vi "display.vi"(8 "error in (no error)":errorcluster, 11 "GeneralDisplay in":refnum<class "GeneralDisplay.lvclass">) -> (0 "error out":errorcluster, 3 "GeneralDisplay out":refnum<class "GeneralDisplay.lvclass">)   [LabVIEW 2018, in "GeneralDisplay.lvclass"]
uses:
  GeneralDisplay.lvclass
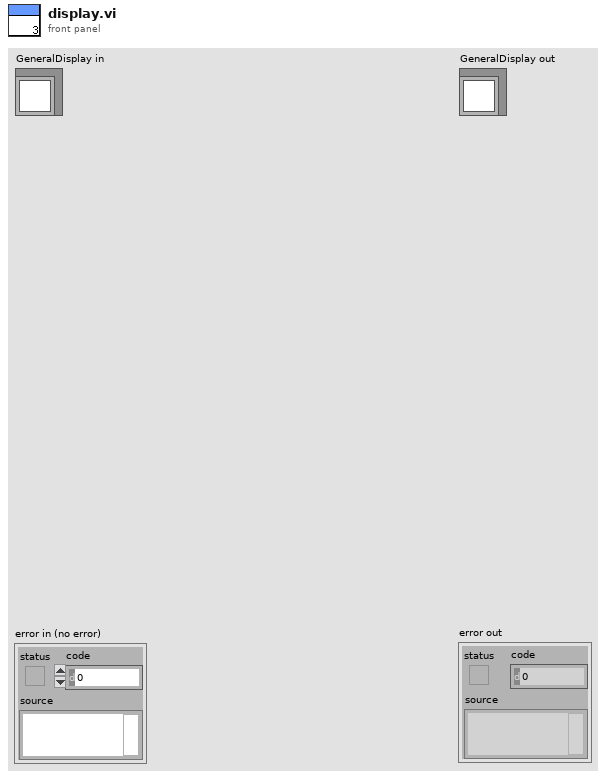
[diagram p1: front panel]
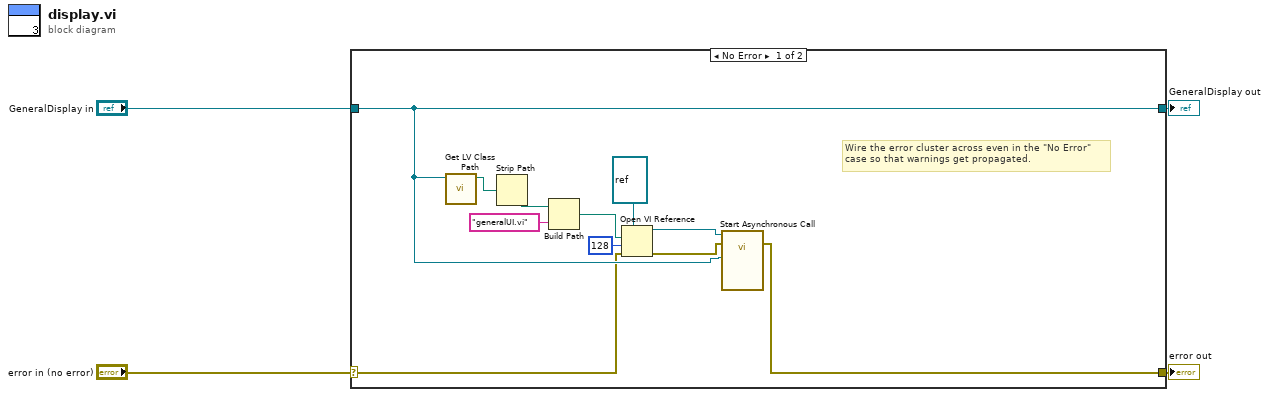
[diagram p0: block diagram]
diagram:
  n1 = case shown="No Error" "error in (no error)" {
    selector: "error in (no error)" -> [w6 w17]
    tunnel: [w5 w17] -> w3
    tunnel: [w7 w16] -> w1
    tunnel: "GeneralDisplay in" -> [w7 w16]
    frame No Error {
      # "Wire the error cluster across even in the \"No Error\"\ncase so that warnings get propagated."
      n2 = call <vilib>:"Get LV Class Path.vi"("object"=w7) -> ("class path"=w15:path)  [unwired: 9 in, 1 out]
      n3 = Strip Path(path=w15) -> (stripped path=w8:path)  [unwired: 1 out]
      n4 = Build Path(base path=w8, name or relative path="generalUI.vi") -> (appended path=w13:path)
      n5 = Open VI Reference(type specifier VI Refnum (for type only)=refnum<vi> refnum, vi path=w13, options=128, error in (no error)=w6) -> (vi reference=w11:refnum<vi>, error out=w10:errorcluster)  [unwired: 2 in]
      n6 = call-by-ref "Start Asynchronous Call"(reference=w11, error in=w10, "GeneralDisplay in"=w7) -> (error out=w5:errorcluster)  [unwired: 11 in, 1 out]
    }
    frame Error {
    }
  }
  "error out" <- w3
  "GeneralDisplay out" <- w1
